vi "MoveTarget.vi"(8 "error in (no error)":errorcluster, 10 "New Target":T1, 11 "3D Scene in":refnum<class "3D Scene.lvclass">) -> (0 "error out":errorcluster, 3 "3D Scene out":refnum<class "3D Scene.lvclass">)   [LabVIEW 2015, in "3D Scene.lvclass"]
uses:
  3D Scene.lvclass
  <vilib>/Utility/miscctls.llb/LV3DPointTypeDef.ctl
  3D Scene.lvclass/3D Scene.ctl
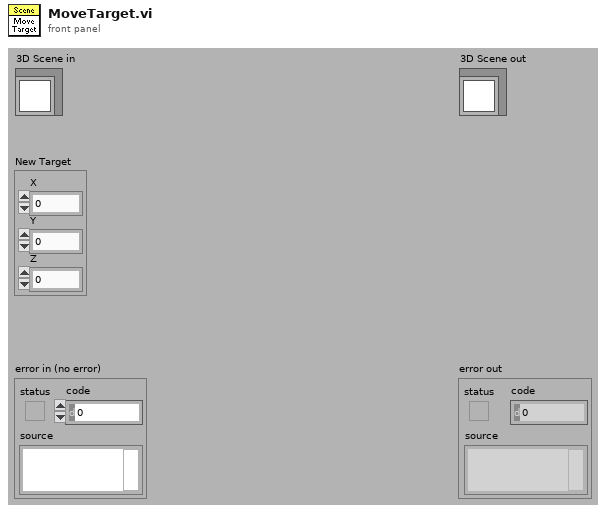
[diagram p1: front panel]
types:
  T1 = typedef "LV3DPointTypeDef.ctl" = cluster{"X":sgl, "Y":sgl, "Z":sgl}
  T2 = typedef "3D Scene.lvclass/3D Point.ctl" = cluster{"X":sgl, "Y":sgl, "Z":sgl}
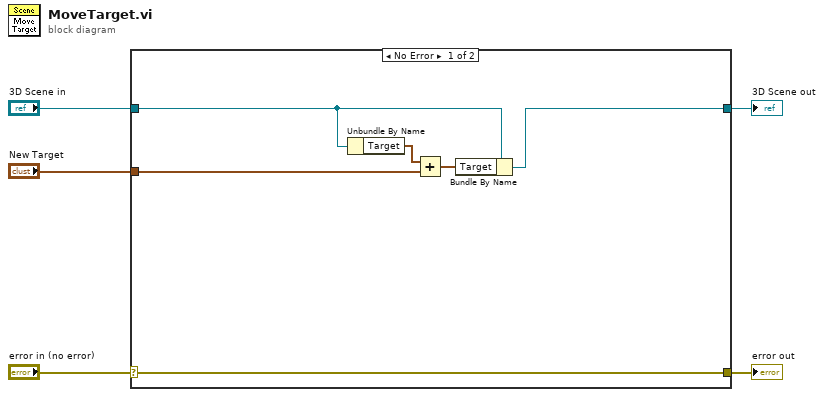
[diagram p0: block diagram]
diagram:
  n1 = case shown="No Error" "error in (no error)" {
    selector: "error in (no error)" -> [w11 w13]
    tunnel: [w11 w13] -> w4
    tunnel: [w10 w12] -> w2
    tunnel: "3D Scene in" -> [w9 w12]
    tunnel: "New Target" -> [w6 _]
    frame No Error {
      n2 = Unbundle By Name(w9) -> ("Target"=w8:T2)
      n3 = Add(x=w8, y=w6) -> (x+y=w7:T2)
      n4 = Bundle By Name(cluster=w9, "Target"=w7) -> (w10:refnum<class "3D Scene.lvclass">)
    }
    frame Error {
    }
  }
  "error out" <- w4
  "3D Scene out" <- w2
